vi "Voltage Ramp Act.vi"(0 "command text in":string[](array[string])) -> ()   [LabVIEW 2025]
doc: "Author: Scott Hannahs <sth@magnet.fsu.edu>\n\nThis software is licensed for use under the “MIT License\"\nCopyright (c) 2025 Scott Hannahs, sth@sth@magnet.sthnet.net\n\nPermission is hereby granted, free of charge, to any person obtaining a copy of this software and associated documentation files (the \"Software\"), to deal in the Software without restriction, including without limitation the rights to use, copy, modify, merge, publish, distribute, sublicense, and/or sell copies of the Software, and to permit persons to whom the Software is furnished to do so, subject to the following conditions: The above copyright notice and this permission notice shall be included in all copies or substantial portions of the Software.\n\nTHE SOFTWARE IS PROVIDED \"AS IS\", WITHOUT WARRANTY OF ANY KIND, EXPRESS OR IMPLIED, INCLUDING BUT NOT LIMITED TO THE WARRANTIES OF MERCHANTABILITY, FITNESS FOR A PARTICULAR PURPOSE AND NONINFRINGEMENT. IN NO EVENT SHALL THE AUTHORS OR COPYRIGHT HOLDERS BE LIABLE FOR ANY CLAIM, DAMAGES OR OTHER LIABILITY, WHETHER IN AN ACTION OF CONTRACT, TORT OR OTHERWISE, ARISING FROM, OUT OF OR IN CONNECTION WITH THE SOFTWARE OR THE USE OR OTHER DEALINGS IN THE SOFTWARE."
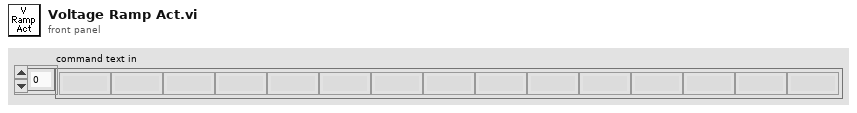
[diagram p1: front panel]
types:
  T1 = typedef "VoltageRamp.ctl" = cluster{"VISA Resource Name":refnum<visa-resource-name>, "extra wait":i32, "start":dbl, "end":dbl, "Sweep Time (H:M:S)":dbl, "Log Linear":bool, "interval(sec)":dbl, "Select instrument":T2}
  T2 = typedef "VoltageRamp Instrument.ctl" = enum16{"Yokogawa GS200 Coarse", "Keithley 24xx Coarse", "Keithley 230"}
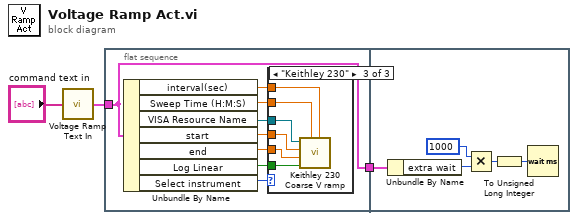
[diagram p0: block diagram]
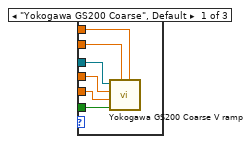
[diagram p2: hidden frame]
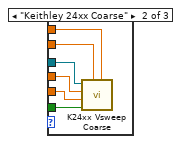
[diagram p3: hidden frame]
diagram:
  n1 = call "Voltage Ramp Text In.vi"("command text in"="command text in") -> ("VoltageRamp"=w2:T1)
  n2 = flat-sequence {
    tunnel: w2 -> [w6]
    tunnel: [w6] -> w1
    tunnel: w1 -> [w31]
    frame #0 {
      n3 = Unbundle By Name(w6) -> ("interval(sec)"=w5:dbl, "Sweep Time (H:M:S)"=w4:dbl, "VISA Resource Name"=w10:refnum<visa-resource-name>, "start"=w9:dbl, "end"=w8:dbl, "Log Linear"=w7:bool, "Select instrument"=w11:T2)
      n4 = case shown="\"Keithley 230\"" w11 {
        tunnel: w10 -> [w17 w23 w29]
        tunnel: w9 -> [w16 w22 w28]
        tunnel: w8 -> [w15 w21 w27]
        tunnel: w7 -> [w14 w20 w26]
        tunnel: w5 -> [w13 w19 w25]
        tunnel: w4 -> [w12 w18 w24]
        frame "Yokogawa GS200 Coarse", Default {
          n5 = call "Yokogawa GS200 Coarse V ramp.vi"("Time Interval (sec)"=w13, "Sweep Time (H:M:S)"=w12, "Mapping"=w14, "End Voltage (V)"=w15, "Start Voltage (V)"=w16, "Yokogawa GS200 Address"=w17) -> ()  [unwired: 5 in, 1 out]
        }
        frame "Keithley 24xx Coarse" {
          n6 = call "K24xx Vsweep Coarse.vi"("Time Interval (sec)"=w19, "Sweep Time (H:M:S)"=w18, "Mapping"=w20, "End Voltage (V)"=w21, "Start Voltage (V)"=w22, "Keithley 24XX Address"=w23) -> ()  [unwired: 5 in, 1 out]
        }
        frame "Keithley 230" {
          n7 = call "Keithley 230 Coarse V ramp.vi"("Time Interval (sec)"=w25, "Sweep Time (H:M:S)"=w24, "Mapping"=w26, "End Voltage (V)"=w27, "Start Voltage (V)"=w28, "Keithley 230 Address"=w29) -> ()  [unwired: 5 in, 1 out]
        }
      }
    }
    frame #1 {
      n8 = Unbundle By Name(w31) -> ("extra wait"=w30:i32)
      n9 = Multiply(x=1000 ("y"), y=w30) -> (x*y=w33:i32)
      n10 = To Unsigned Long Integer(number=w33) -> (unsigned 32bit integer=w32:u32)
      n11 = Wait (ms)(milliseconds to wait=w32) -> ()  [unwired: 1 out]
    }
  }
